vi "TestFFTOrder.vi"(8 "振动判定":T1, 9 "振动判定范围":T2, 10 "spectrum info":T3[](array[typedef]) {"x-axis units" items=["Time (s)"=0, "Frequency-CB (Hz)"=1, "Frequency-CPB (Hz)"=1248, "Frequency-Arbitrary (Hz)"=2357, "Quefrency (s)"=2, "Revolutions (rev)"=3, "Order"=4, "Speed (RPM)"=11, "Speed (rad/s)"=21, "Index"=65535]; "weighting filter" items=["Linear", "A-weighting", "B-weighting", "C-weighting", "ITU-R 468-4", "Dolby", "CCITT", "C-message", "Wb", "Wc", "Wd", "We", "Wf", "Wh", "Wj", "Wk", "Wm", "AES17 20 kHz lowpass", "AES17 40 kHz lowpass", "AES17 20 kHz highpass", "AES17 40 kHz highpass"]; "dB reference [EU]" format="%.2f"; "engineering units" items=["custom..."=0, "V"=1, "A"=21, "C"=30, "pC"=31, "s"=32, "-"=29, "Pa"=2, "N"=20, "g"=3, "m/s^2"=4, "m/s"=5, "m"=6, "mm/s"=12, "mm"=13, "micron/s"=14, "micron"=15, "in/s^2"=7, "in/s"=8, "in"=9, "mil/s"=10, "mil"=11, "rad/s^2"=16, "rad/s"=17, "rad"=18, "deg/s^2"=26, "deg/s"=27, "deg"=28, "RPM"=22, "cycle/s^2"=23, "Hz"=24, "cycle"=25, "strain"=19]; "spectral info"."window" items=["None "=0, "Hanning"=1, "Hamming"=2, "Blackman-Harris"=3, "Exact Blackman"=4, "Blackman"=5, "Flat Top"=6, "4 Term B-Harris "=7, "7 Term B-Harris"=8, "Low Sidelobe"=9, "Force - Exponential"=10, "Gaussian"=62]}, 11 "FFT 5":cluster{"x0":dbl, "dx":dbl, "Y":dbl[]}[](graph) caption="spectrum") -> (1 "数组":cluster{"freq.":dbl, "dB":dbl}[][](array[cluster]), 2 "Test Result":bool[](array[boolean]), 3 "FFT 2":cluster{"x0":dbl, "dx":dbl, "Y":dbl[]}[](graph))   [LabVIEW 2020]
uses:
  <vilib>/_NISVFA/_Shared subVIs/Controls/svc_Spectrum Info.ctl
  <vilib>/_NISVFA/_Shared subVIs/Controls/svc_X-Axis Units.ctl
  <vilib>/_NISVFA/_Shared subVIs/Controls/svc_Spectrum Type.ctl
  <vilib>/_NISVFA/_Shared subVIs/Controls/svc_Engineering Units Text Ring.ctl
  <vilib>/_NISVFA/_Shared subVIs/Controls/svc_Weighting Filter Text Ring.ctl
  <vilib>/_NISVFA/_Shared subVIs/Controls/svc_Complimentary Spectrum Units.ctl
  <vilib>/_NISVFA/_Spectrum Processing/SVFA Get Spectrum Subset (1 Ch).vi
  <vilib>/_NISVFA/_Spectrum Processing/SVFA Spectrum Peak Search (1 Ch).vi
  <vilib>/_NISVFA/_Shared subVIs/Common/svc_Spectrum Units.vi
  <vilib>/_NISVFA/_Spectrum Processing/subVIs/svfa_Spectrum Peak Search.vi
  <vilib>/_NISVFA/_Spectrum Processing/subVIs/svfa_Peak Rough Search Indices.vi
  <vilib>/measure/mamon.llb/Create Continuous Mask.vi
  <vilib>/_NISVFA/_Shared subVIs/Common/svc_Format Value (DBL).vi
  <vilib>/_NISVFA/_Shared subVIs/Common/svc_Engineering Units to Unit Label.vi
  <vilib>/_NISVFA/_Shared subVIs/Common/svc_Unit Label Lexical Class.vi
  <vilib>/_NISVFA/_Shared subVIs/Common/svc_Get Weighting Enum and Labels.vi
  <vilib>/_NISVFA/_Shared subVIs/Common/svc_Check Frequency Range in Spectrum.vi
  <vilib>/_NISVFA/_Shared subVIs/Common/svc_Caller VI Returned in Error Source.vi
  <vilib>/_NISVFA/_Shared subVIs/Common/svc_Convert Frequency to Frequency String.vi
  <vilib>/_NISVFA/_Shared subVIs/Common/svc_Build Unit Label for Frequency Range.vi
  <vilib>/_NISVFA/_Spectrum Processing/subVIs/svfa_Three Finger Peak Search.vi
  <vilib>/measure/mamon.llb/Limit Testing Frequency.vi
  <vilib>/measure/NI_MAPro.lvlib
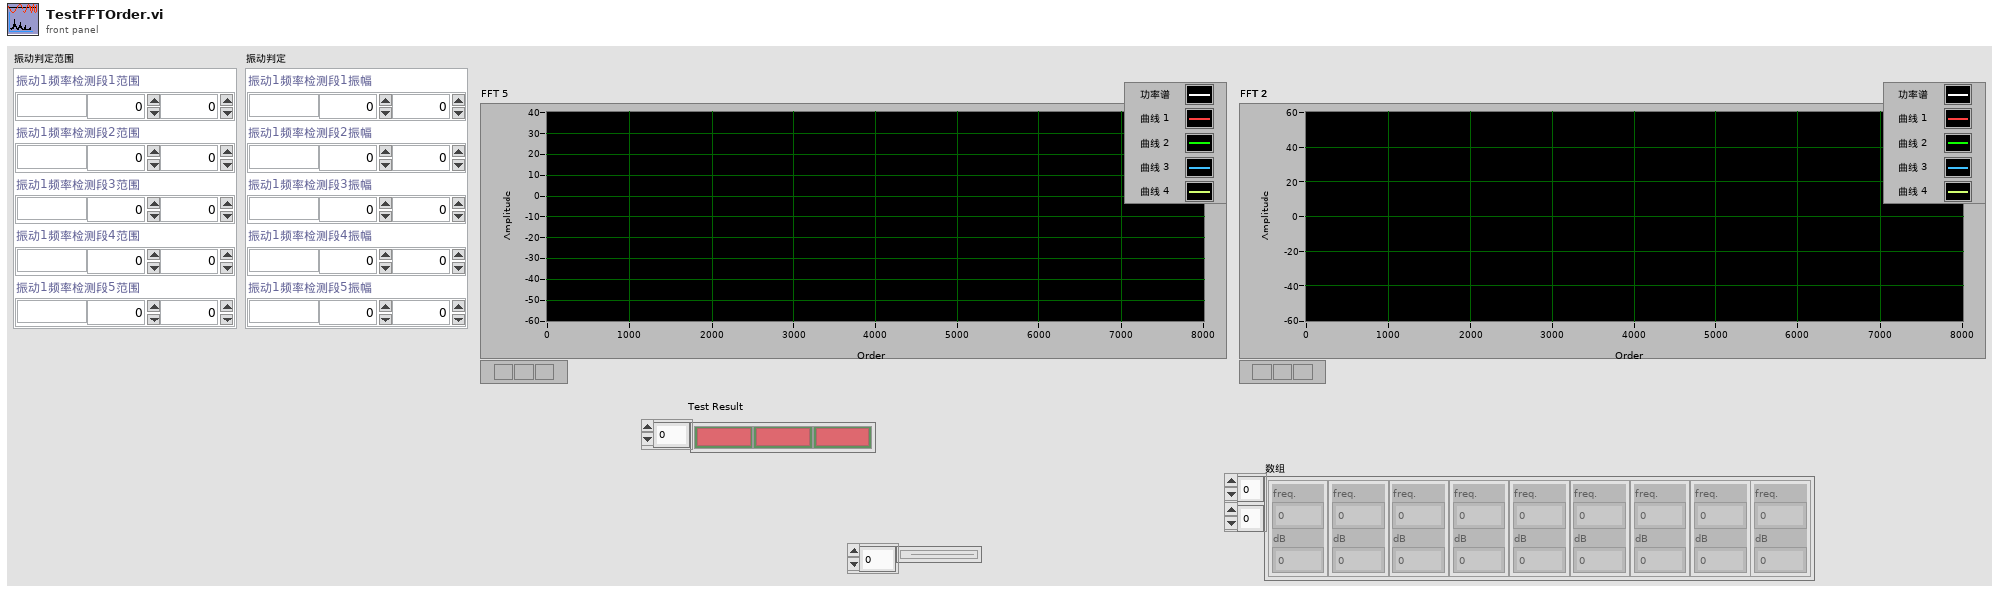
[diagram p1: front panel]
types:
  T1 = cluster{"振动1频率检测段1振幅":cluster{"单位":string, "下限":dbl, "上限":dbl}, "振动1频率检测段2振幅":cluster{"单位":string, "下限":dbl, "上限":dbl}, "振动1频率检测段3振幅":cluster{"单位":string, "下限":dbl, "上限":dbl}, "振动1频率检测段4振幅":cluster{"单位":string, "下限":dbl, "上限":dbl}, "振动1频率检测段5振幅":cluster{"单位":string, "下限":dbl, "上限":dbl}}
  T2 = cluster{"振动1频率检测段1范围":cluster{"单位":string, "下限":dbl, "上限":dbl}, "振动1频率检测段2范围":cluster{"单位":string, "下限":dbl, "上限":dbl}, "振动1频率检测段3范围":cluster{"单位":string, "下限":dbl, "上限":dbl}, "振动1频率检测段4范围":cluster{"单位":string, "下限":dbl, "上限":dbl}, "振动1频率检测段5范围":cluster{"单位":string, "下限":dbl, "上限":dbl}}
  T3 = typedef "svc_Spectrum Info.ctl" = cluster{"channel name":string, "description":string, "x-axis units":T4, "spectral info":cluster{"spectrum type":T5, "linear/dB":enum16{"linear", "dB"}, "window":u16, "window size":i32, "FFT size":i32}, "engineering units":T6, "custom label":string, "dB reference [EU]":dbl, "peak units":enum16{"rms", "peak", "peak-peak"}, "weighting filter":T7, "spectral density?":bool, "unit label":string, "spectrum skewed?":bool, "complimentary spectrum units":T8}
  T4 = typedef "svc_X-Axis Units.ctl" = u16
  T5 = typedef "svc_Spectrum Type.ctl" = enum16{"FFT Spectrum [complex]", "Amplitude [Magnitude]", "Power [Magnitude^2]", "Cross Spectrum [complex]", "Frequency Response [Complex]"}
  T6 = typedef "svc_Engineering Units Text Ring.ctl" = u16
  T7 = typedef "svc_Weighting Filter Text Ring.ctl" = u16
  T8 = typedef "svc_Complimentary Spectrum Units.ctl" = enum16{"none", "radians", "degrees", "cycles", "imaginary"}
  T9 = cluster{"single/multiple":enum16{"Multiple Peaks", "Single Max Peak"}, "threshold":dbl}
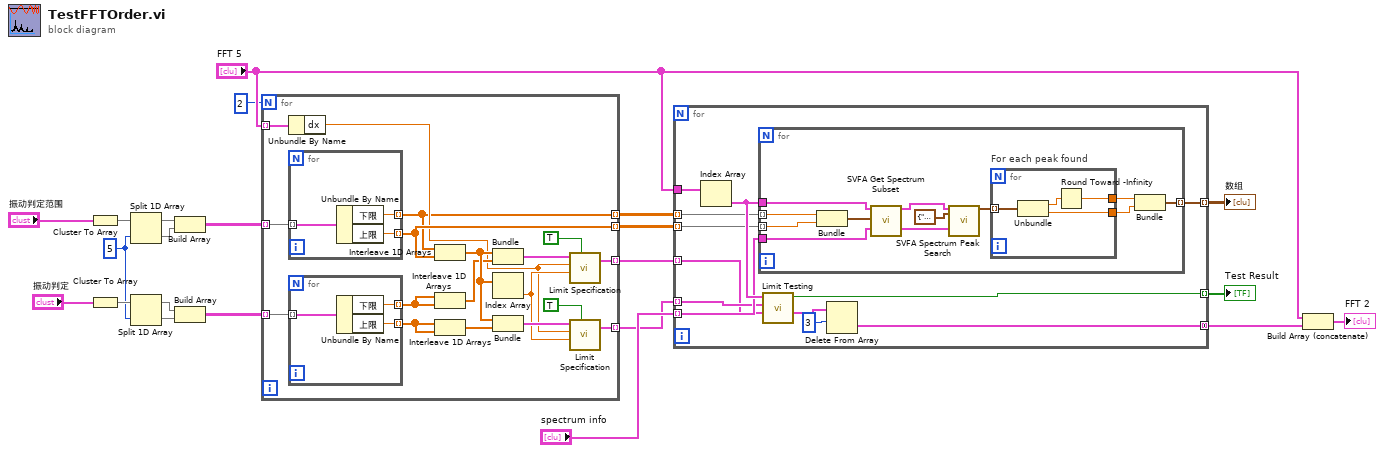
[diagram p0: block diagram]
diagram:
  w18 = 5 ("索引")
  n1 = Cluster To Array(cluster="振动判定范围") -> (array=w20:cluster{"单位":string, "下限":dbl, "上限":dbl}[])
  n2 = Cluster To Array(cluster="振动判定") -> (array=w19:cluster{"单位":string, "下限":dbl, "上限":dbl}[])
  n3 = Split 1D Array(array=w20, index=w18) -> (first subarray=w17:cluster{"单位":string, "下限":dbl, "上限":dbl}[], second subarray=w16:cluster{"单位":string, "下限":dbl, "上限":dbl}[])
  n4 = Split 1D Array(array=w19, index=w18) -> (first subarray=w15:cluster{"单位":string, "下限":dbl, "上限":dbl}[], second subarray=w14:cluster{"单位":string, "下限":dbl, "上限":dbl}[])
  n5 = Build Array(w17, w16) -> (w13:cluster{"单位":string, "下限":dbl, "上限":dbl}[][])
  n6 = Build Array(w15, w14) -> (w12:cluster{"单位":string, "下限":dbl, "上限":dbl}[][])
  n7 = for {
    N: 2 -> [_]
    tunnel: w13 -> [w39] mode=indexing
    tunnel: w12 -> [w38] mode=indexing
    tunnel: [w40] -> w7 mode=indexing
    tunnel: [w34] -> w8 mode=indexing
    tunnel: [w26] -> w6 mode=indexing
    tunnel: "FFT 5" -> [w25] mode=indexing
    tunnel: [w23] -> w1 mode=indexing
    n8 = Unbundle By Name(w25) -> ("dx"=w24:dbl)
    n9 = for {
      tunnel: w39 -> [w46] mode=indexing
      tunnel: [w45] -> w23 mode=indexing
      tunnel: [w44] -> w26 mode=indexing
      n10 = Unbundle By Name(w46) -> ("下限"=w45:dbl, "上限"=w44:dbl)
    }
    n11 = for {
      tunnel: w38 -> [w43] mode=indexing
      tunnel: [w42] -> w37 mode=indexing
      tunnel: [w41] -> w27 mode=indexing
      n12 = Unbundle By Name(w43) -> ("下限"=w42:dbl, "上限"=w41:dbl)
    }
    n13 = Interleave 1D Arrays(w23, w26) -> (w32:dbl[])
    n14 = Interleave 1D Arrays(w37, w37) -> (w31:dbl[])
    n15 = Interleave 1D Arrays(w27, w27) -> (w33:dbl[])
    n16 = Bundle(w32, w31) -> (w35:cluster{dbl[], dbl[]})  [unwired: 1 in]
    n17 = Index Array(array=w32) -> (element=w30:dbl)  [unwired: 1 in]
    n18 = Bundle(w32, w33) -> (w36:cluster{dbl[], dbl[]})  [unwired: 1 in]
    n19 = call-poly <vilib>:"Limit Specification.vi"("Specification Cluster"=w35, "dx"=w24, "x0"=w30, "Reset"=TRUE) -> ("Limit"=w34:cluster{"x0":dbl, "dx":dbl, "Y":dbl[]})  [unwired: 1 in, 1 out]
    n20 = call-poly <vilib>:"Limit Specification.vi"("Specification Cluster"=w36, "dx"=w24, "x0"=w30, "Reset"=TRUE) -> ("Limit"=w40:cluster{"x0":dbl, "dx":dbl, "Y":dbl[]})  [unwired: 1 in, 1 out]
  }
  n21 = for {
    tunnel: [w57] -> w11 mode=indexing
    tunnel: [w47] -> w10 mode=indexing
    tunnel: "FFT 5" -> [w56]
    tunnel: "spectrum info" -> [w55] mode=indexing
    tunnel: w8 -> [w49] mode=indexing
    tunnel: w7 -> [w54] mode=indexing
    tunnel: w6 -> [w53] mode=indexing
    tunnel: [w50] -> w5 mode=concatenating
    tunnel: w1 -> [w48] mode=indexing
    n22 = Index Array(array=w56) -> (element=w58:cluster{"x0":dbl, "dx":dbl, "Y":dbl[]})  [unwired: 1 in]
    n23 = for {
      tunnel: w58 -> [w70]
      tunnel: w55 -> [w69]
      tunnel: w53 -> [w61] mode=indexing
      tunnel: [w64] -> w57 mode=indexing
      tunnel: w48 -> [w59] mode=indexing
      n24 = Bundle("下限"=w59, "上限"=w61) -> (w68:cluster{"下限":dbl, "上限":dbl})  [unwired: 1 in]
      n25 = call-poly <vilib>:"SVFA Get Spectrum Subset.vi"("spectrum"=w70, "range"=w68, "spectrum info"=w69) -> ("spectrum subset"=w60:cluster{"x0":dbl, "dx":dbl, "magnitude":dbl[]}, "dup spectrum info"=w63:T3)  [unwired: 11 in, 4 out]
      n26 = call-poly <vilib>:"SVFA Spectrum Peak Search.vi"("spectrum"=w60, "peak search settings"=T9 {"single/multiple"=enum."Single Max Peak", "threshold"=0.0}, "spectrum info in"=w63) -> ("peaks"=w66:cluster{"freq. or order":dbl, "value":dbl}[])  [unwired: 12 in, 4 out]
      n27 = for "For each peak found" {
        tunnel: w66 -> [w74] mode=indexing
        tunnel: [w72] -> w65
        tunnel: [w73] -> w62
        n28 = Unbundle(w74) -> ("freq. or order"=w71:dbl, "value"=w73:dbl)
        n29 = Round Toward -Infinity(1:w71) -> (0:w72:dbl)
      }
      n30 = Bundle(w65, "value"=w62) -> (w64:cluster{dbl, "value":dbl})  [unwired: 1 in]
    }
    n31 = call-poly <vilib>:"Limit Testing.vi"("lower limit"=w49, "upper limit"=w54, "signal in"=w58) -> ("output values"=w52:cluster{"x0":dbl, "dx":dbl, "Y":dbl[]}[], "test passed?"=w47:bool)  [unwired: 3 in, 4 out]
    n32 = Delete From Array(array=w52, length=3 ("长度")) -> (deleted portion=w50:cluster{"x0":dbl, "dx":dbl, "Y":dbl[]}[])  [unwired: 1 in, 1 out]
  }
  "数组" <- w11
  "Test Result" <- w10
  n33 = Build Array (concatenate)("FFT 5", w5) -> (→"FFT 2":cluster{"x0":dbl, "dx":dbl, "Y":dbl[]}[])
